vi "Global Coeff corr H1.vi"() -> ()   [LabVIEW 2016]
panel:
  in  "H1 H2 CORR":dbl[](array[numeric])
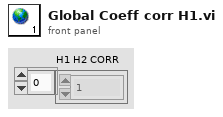
[diagram p1: front panel]
diagram:
